vi "Pump Start Detect Attempt (RT).vi"() -> ()   [LabVIEW 2019]
panel:
  out "Detected Starts":u32[](array[numeric])
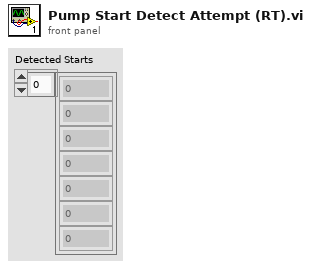
[diagram p1: front panel]
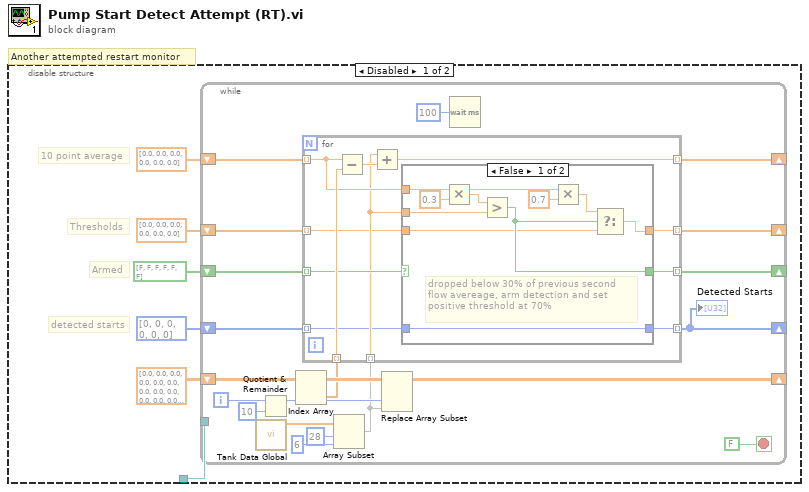
[diagram p0: block diagram]
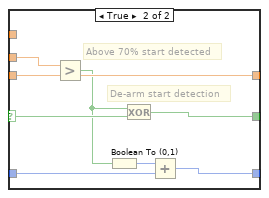
[diagram p2: hidden frame]
diagram:
  # "Another attempted restart monitor"
  n1 = disable-structure shown="Disabled" {
    disable-tunnel: _ -> [w6 _]
    frame Disabled {
      # "Armed"
      # "Thresholds"
      # "detected starts"
      # "10 point average"
      n2 = while {
        tunnel: w6 -> [_]
        shift-right: [w17] -> _
        shift-left: dbl[][] [[0.0, 0.0, 0.0, 0.0, 0.0, 0.0, 0.0, 0.0, 0.0, 0.0], [0.0, 0.0, 0.0, 0.0, 0.0, 0.0, 0.0, 0.0, 0.0, 0.0], [0.0, 0.0, 0.0, 0.0, 0.0, 0.0, 0.0, 0.0, 0.0, 0.0], [0.0, 0.0, 0.0, 0.0, 0.0, 0.0, 0.0, 0.0, 0.0, 0.0], [0.0, 0.0, 0.0, 0.0, 0.0, 0.0, 0.0, 0.0, 0.0, 0.0], [0.0, 0.0, 0.0, 0.0, 0.0, 0.0, 0.0, 0.0, 0.0, 0.0]] -> [w19]
        shift-right: [w12] -> _
        shift-left: dbl[] [0.0, 0.0, 0.0, 0.0, 0.0, 0.0] -> [w13]
        shift-right: [w7] -> _
        shift-left: u32[] [0, 0, 0, 0, 0, 0] -> [w11]
        shift-right: [w8] -> _
        shift-left: dbl[] [0.0, 0.0, 0.0, 0.0, 0.0, 0.0] -> [w14]
        shift-right: [w9] -> _
        shift-left: bool[] [FALSE, FALSE, FALSE, FALSE, FALSE, FALSE] -> [w10]
        i -> [w21]
        stop <- FALSE stop-if-true
        n3 = call "Tank Data Global.vi"() -> ("Tank Data OUT"=w24:dbl[])  [unwired: 11 in]
        n4 = Quotient & Remainder(x=w21, y=10) -> (x-y*floor(x/y)=w18:i32)  [unwired: 1 out]
        n5 = Index Array(array=w19, index (col)=w18) -> (element=w16:dbl[])  [unwired: 1 in]
        n6 = Array Subset(array=w24, index=28, length=6) -> (w15:dbl[])
        n7 = for {
          tunnel: w16 -> [w37] mode=indexing
          tunnel: w15 -> [w32] mode=indexing
          tunnel: w14 -> [w30] mode=indexing
          tunnel: w13 -> [w33] mode=indexing
          tunnel: [w35] -> w12 mode=indexing
          tunnel: w11 -> [w28] mode=indexing
          tunnel: w10 -> [w34] mode=indexing
          tunnel: [w31] -> w9 mode=indexing
          tunnel: [w29] -> w8 mode=indexing
          tunnel: [w27] -> w7 mode=indexing
          n8 = Subtract(x=w33, y=w37) -> (x-y=w36:dbl)
          n9 = Add(x=w32, y=w36) -> (x+y=w35:dbl)
          n10 = case shown="False" w34 {
            selector: w34 -> [_ w50]
            tunnel: w33 -> [w44 _]
            tunnel: w32 -> [w45 w55]
            tunnel: [w42 w48] -> w31
            tunnel: w30 -> [w40 w51]
            tunnel: [w39 w51] -> w29
            tunnel: w28 -> [w38 w53]
            tunnel: [w38 w52] -> w27
            frame False {
              # "dropped below 30% of previous second\nflow avereage, arm detection and set\npositive threshold at 70%"
              n11 = Multiply(x=w44, y=0.3) -> (x*y=w46:dbl)
              n12 = Greater?(x=w46, y=w45) -> (0:w42:bool)
              n13 = Multiply(x=w44, y=0.7) -> (x*y=w41:dbl)
              n14 = Select(t=w41, s=w42, f=w40) -> (s? t:f=w39:dbl)
            }
            frame True {
              # "De-arm start detection"
              # "Above 70% start detected"
              n15 = Greater?(x=w55, y=w51) -> (0:w49:bool)
              n16 = Boolean To (0,1)(Boolean=w49) -> (0, 1=w54:i16)
              n17 = Exclusive Or(1:w50, 2:w49) -> (0:w48:bool)
              n18 = Add(x=w54, y=w53) -> (x+y=w52:u32)
            }
          }
        }
        "Detected Starts" <- w7
        n19 = Replace Array Subset(array=w19, new element=w15, index (col)=w18) -> (w17:dbl[][])  [unwired: 1 in]
        n20 = Wait (ms)(milliseconds to wait=u32 100) -> ()  [unwired: 1 out]
      }
    }
    frame Enabled {
    }
  }
